vi "Forward Packet to Server.vi"(10 "Message":T1, 11 "Session in":refnum<class "Session.lvclass">) -> (0 "error out":errorcluster)   [LabVIEW 2013, in "MQTT Server.lvlib" / "Session.lvclass"]
uses:
  Session.lvclass
  MQTT_Base/Response -- cluster.ctl
  Control Packets/ControlPacket/ControlPacket.lvclass
  Pending ACKs -- cluster.ctl
  Control Packets/ControlPacket/ControlPacket.lvclass/ControlPacket.ctl
  Session.lvclass/Session.ctl
  Connection/TCPConnection.lvclass
  MQTT_Base/MQTT_Base.lvclass
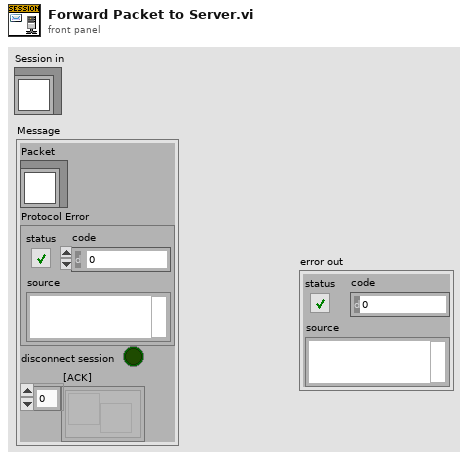
[diagram p1: front panel]
types:
  T1 = typedef "MQTT Server.lvlib/MQTT_Base.lvclass/Response -- cluster.ctl" = cluster{"Packet":refnum<class "ControlPacket.lvclass">, "Protocol Error":errorcluster, "disconnect session":bool, "[ACK]":refnum<notifier>[]}
  T2 = typedef "MQTT Server.lvlib/Session.lvclass/Pending ACKs -- cluster.ctl" = cluster{"Message":refnum<class "ControlPacket.lvclass">, "[ACK]":refnum<notifier>[], "Packet Identifier":u16}
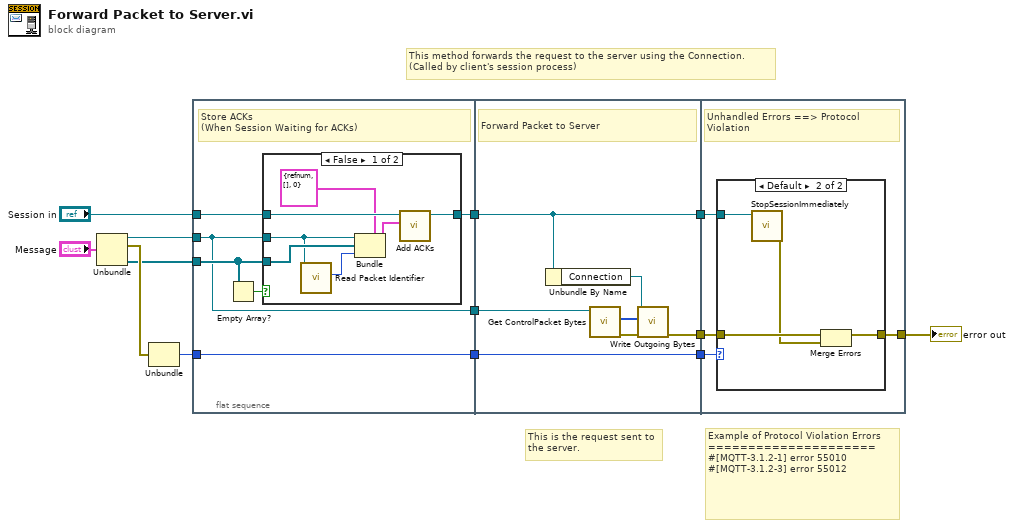
[diagram p0: block diagram]
diagram:
  # "This method forwards the request to the server using the Connection.\n(Called by client's session process)"
  # "This is the request sent to\nthe server."
  # "Example of Protocol Violation Errors\n=====================\n#[MQTT-3.1.2-1] error 55010\n#[MQTT-3.1.2-3] error 55012"
  n1 = Unbundle("Message") -> ("Packet"=w13:refnum<class "ControlPacket.lvclass">, "Protocol Error"=w9:errorcluster, "[ACK]"=w3:refnum<notifier>[])  [unwired: 1 out]
  n2 = Unbundle(w9) -> ("code"=w6:i32)  [unwired: 2 out]
  n3 = flat-sequence {
    tunnel: w6 -> [w19]
    tunnel: "Session in" -> [w18]
    tunnel: w13 -> [w14]
    tunnel: [w19] -> w4
    tunnel: w3 -> [w15]
    tunnel: [w16] -> w2
    tunnel: [w14] -> w1
    tunnel: [w31] -> w8
    tunnel: [w29] -> w7
    tunnel: [w28] -> w5
    tunnel: w4 -> [w29]
    tunnel: w2 -> [w28]
    tunnel: w1 -> [w33]
    tunnel: [w35] -> w11
    tunnel: w8 -> [w36]
    tunnel: w7 -> [w37]
    tunnel: w5 -> [w38]
    frame #0 {
      # "Store ACKs\n(When Session Waiting for ACKs)"
      n4 = Empty Array?(array=w15) -> (empty?=w17:bool)
      n5 = case shown="False" w17 {
        tunnel: w18 -> [w26 w27]
        tunnel: [w25 w27] -> w16
        tunnel: w14 -> [w22 _]
        tunnel: w15 -> [w24 _]
        frame False {
          n6 = call "Read Packet Identifier.vi"("ControlPacket in"=w22) -> ("Packet Identifier"=w21:u16)  [unwired: 9 in, 1 out]
          n7 = Bundle(cluster=T2 {"Message"=refnum, "[ACK]"=[], "Packet Identifier"=0} ("Pending ACK"), "Message"=w22, "[ACK]"=w24, "Packet Identifier"=w21) -> (w23:T2)
          n8 = call "Add ACKs.vi"("Pending ACK"=w23, "Session in"=w26) -> ("Session out"=w25:refnum<class "Session.lvclass">)  [unwired: 8 in, 1 out]
        }
        frame True {
          # "No Acks."
        }
      }
    }
    frame #1 {
      # "Forward Packet to Server"
      n9 = Unbundle By Name(w28) -> ("Connection"=w30:refnum<class "TCPConnection.lvclass">)
      n10 = call "Get ControlPacket Bytes.vi"("ControlPacket"=w33) -> ("error out"=w32:errorcluster, "Bytes Stream"=w34:u8[])  [unwired: 8 in, 1 out]
      n11 = call "Write Outgoing Bytes.vi"("error in (no error)"=w32, "Bytes"=w34, "TCPConnection in"=w30) -> ("error out"=w31:errorcluster)  [unwired: 7 in, 1 out]
    }
    frame #2 {
      # "Unhandled Errors ==> Protocol Violation"
      n12 = case shown="Default" w37 {
        tunnel: w38 -> [_ w43]
        tunnel: w36 -> [w39 w42]
        tunnel: [w39 w40] -> w35
        frame 0 {
        }
        frame Default {
          n13 = call "StopSessionImmediately.vi"("Session in"=w43) -> ("error out"=w41:errorcluster)  [unwired: 9 in, 1 out]
          n14 = Merge Errors(w42, w41) -> (w40:errorcluster)
        }
      }
    }
  }
  "error out" <- w11
